vi "VT4001_Chamber Close.vi"(8 "error in":errorcluster, 11 "VISA Resource":refnum<visa-resource-name>) -> (0 "error out":errorcluster={"status"=FALSE, "code"=1073676294, "source"="VISA Read in MB Master.lvlib:MB_ADU_RTU.lvclass:RX ADU.vi:4960001->MB Master.lvlib:MB_Master_Serial.lvclass:Querry.vi:3550001->MB Master.lvlib:Write Single Coil.vi:160001->VT4001_Chamber Close.vi"}, 2 "OK":bool=TRUE)   [LabVIEW 2019]
doc: "Modbus Comm Tester\n\nThis VI demonstrates the usage of the Modbus Master API for both TCP and Serial connections.\nIt is also a useful tool for testing communication with your modbus device. You can test different\ncommunication parameters and coil/register address ranges without having to write any code.\n\nCopyright (c) 2016, Plasmionique Inc.\nAll rights reserved.\n\nLicense: BSD (2-Clause) - http://opensource.org/licenses/BSD-2-Clause"
uses:
  <vilib>/Plasmionique/MB Master/MB_Master_Serial/MB_Master_Serial.lvclass
  D:/National Instruments/LabVIEW 2019/vi.lib/Plasmionique/MB Master/MB_Master/MB_Master.lvclass
  <vilib>/Plasmionique/MB Master/MB Master.lvlib
panel:
  # "Communication Settings"
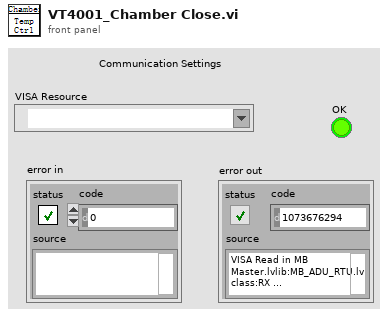
[diagram p1: front panel]
types:
  T1 = cluster{"baud rate (bps)":u32, "stop bits":u16, "parity":u16, "flow control":u16, "timeout":u32, "retries":i32}
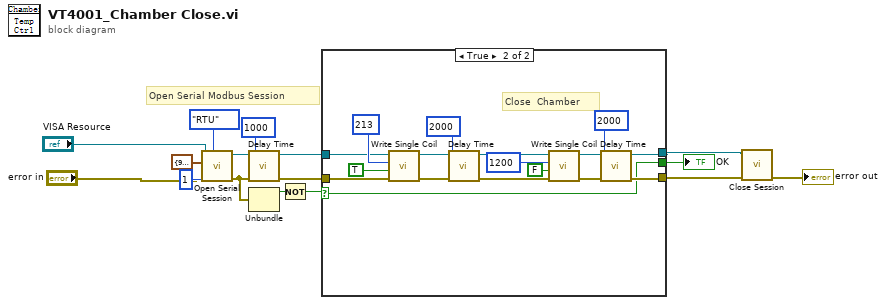
[diagram p0: block diagram]
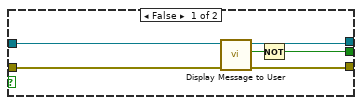
[diagram p2: hidden frame]
diagram:
  # "Open Serial Modbus Session"
  n1 = call <vilib>:"Open Serial Session.vi"("Mode (RTU)"=enum16{"RTU", "ASCII"}."RTU", "Error in"="error in", "Slave ID"=u8 1, "Serial Config"=T1 {"baud rate (bps)"=9600, "stop bits"=10, "parity"=0, "flow control"=0, "timeout"=1000, "retries"=1}, "VISA Resource"="VISA Resource") -> ("Error out"=w12:errorcluster, "MB_Serial session"=w13:refnum<class "MB_Master_Serial.lvclass">)  [unwired: 5 in]
  n2 = call "Delay Time.vi"("Error In"=w12, "Delay Time (ms)"=u32 1000) -> ("Error Out"=w11:errorcluster)  [unwired: 9 in]
  n3 = Unbundle(w12) -> ("status"=w15:bool)  [unwired: 2 out]
  n4 = Not(x=w15) -> (.not. x?=w14:bool)
  n5 = case shown="True" w14 {
    selector: w14 -> [_ w29]
    tunnel: w13 -> [w16 w22]
    tunnel: w11 -> [w20 w23]
    tunnel: [w19 w30] -> w4
    tunnel: [w17 w29] -> w10
    tunnel: [w16 w31] -> w5
    frame False {
      n6 = call "Display Message to User"("error in (no error)"=w20) -> ("error out"=w19:errorcluster, "OK"=w18:bool)  [unwired: 9 in]
      n7 = Not(x=w18) -> (.not. x?=w17:bool)
    }
    frame True {
      # "Close  Chamber"
      n8 = call <vilib>:"Write Single Coil.vi"("error in (no error)"=w23, "value"=TRUE, "address"=u16 213, "MB session in"=w22) -> ("error out"=w24:errorcluster, "MB session out"=w21:refnum<class "MB_Master_Serial.lvclass">)  [unwired: 6 in]
      n9 = call "Delay Time.vi"("Error In"=w24, "Delay Time (ms)"=u32 2000) -> ("Error Out"=w25:errorcluster)  [unwired: 9 in]
      n10 = call <vilib>:"Write Single Coil.vi"("error in (no error)"=w25, "value"=FALSE, "address"=u16 1200, "MB session in"=w21) -> ("error out"=w33:errorcluster, "MB session out"=w31:refnum<class "MB_Master_Serial.lvclass">)  [unwired: 6 in]
      n11 = call "Delay Time.vi"("Error In"=w33, "Delay Time (ms)"=u32 2000) -> ("Error Out"=w30:errorcluster)  [unwired: 9 in]
    }
  }
  "OK" <- w10
  n12 = call-dynamic "Close Session.vi"("error in (no error)"=w4, "MB_Serial session"=w5) -> ("error out"=→"error out":errorcluster)  [unwired: 9 in]
